vi "Initialize Test Fixture.vi"(11 "Serial Number":string) -> (0 "error out":errorcluster)   [LabVIEW 2013]
uses:
  <instrlib>/Driver Simulation/Fixture.lvlib
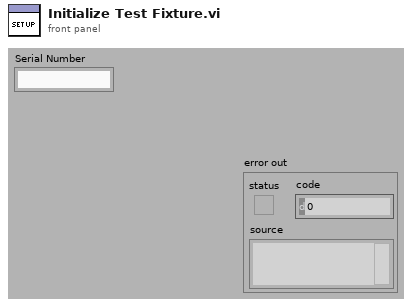
[diagram p1: front panel]
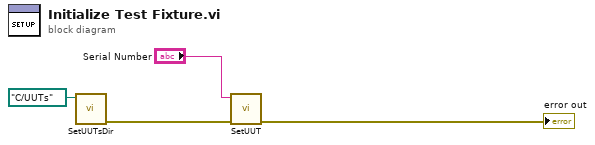
[diagram p0: block diagram]
diagram:
  n1 = call <instrlib>:"SetUUTsDir.vi"("UUTDirectory"=path "C:/UUTs") -> ("error out"=w2:errorcluster)  [unwired: 10 in]
  n2 = call <instrlib>:"SetUUT.vi"("error in (no error)"=w2, "Serial Number"="Serial Number") -> ("error out"=→"error out":errorcluster)  [unwired: 9 in]
